vi "Configure Dialog.vi"(8 "Error In":errorcluster, 11 "Save SV to Library Msg in":refnum<class "Save SV to Library Msg.lvclass">) -> (0 "Error Out":errorcluster, 2 "OK?":bool, 3 "Save SV to Library Msg out":refnum<class "Save SV to Library Msg.lvclass">)   [LabVIEW 2014, in "CS++DSCManager.lvlib" / "Save SV to Library Msg.lvclass"]
doc: "This overrides of this dynamic dispatch VI open the frontpanel to set derived message attributes."
uses:
  Save SV to Library Msg.lvclass
  Save SV to Library Msg.lvclass/Save SV to Library Msg.ctl
panel:
  in  "OK":bool
  in  "Cancel":bool
  in  "Library Path":path
  in  "Shared Variables":refnum<k21>[](array[refnum])
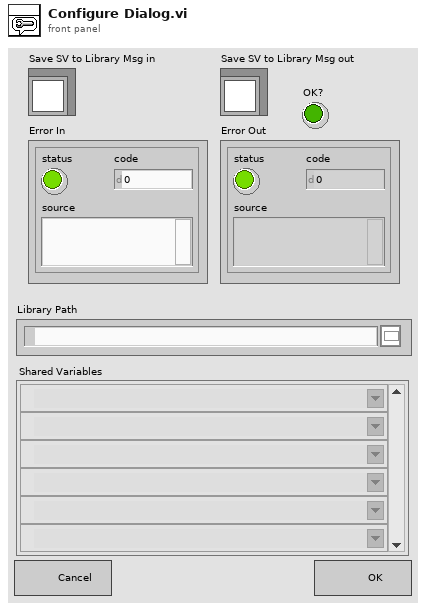
[diagram p1: front panel]
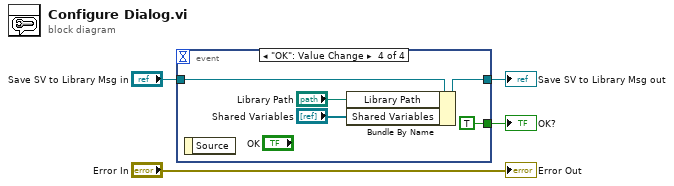
[diagram p0: block diagram]
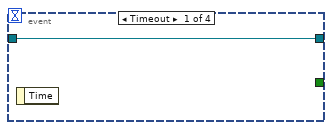
[diagram p2: hidden frame]
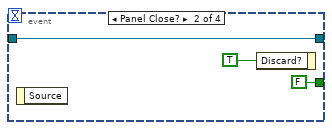
[diagram p3: hidden frame]
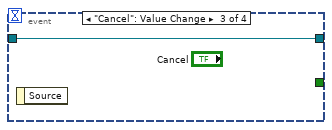
[diagram p4: hidden frame]
diagram:
  n1 = event shown="[3] \"OK\": Value Change" {
    selector: _ -> [_ _ _ _]
    dyn-events: _ -> [_ _ _ _]
    timeout: _ -> [_ _ _ _]
    tunnel: [w5 w6 w9 w13] -> w2
    tunnel: "Save SV to Library Msg in" -> [w5 w6 w9 w14]
    tunnel: [_ FALSE _ TRUE] -> w1
    event Timeout {
      n2 = event-data() -> ()  [unwired: 1 in, 1 out]
    }
    event Panel Close? {
      n3 = event-data() -> ()  [unwired: 1 in, 1 out]
      n4 = event-data("Discard?"=TRUE) -> ()  [unwired: 1 in, 1 out]
    }
    event "Cancel": Value Change {
      n5 = event-data() -> ()  [unwired: 1 in, 1 out]
    }
    event "OK": Value Change {
      n6 = event-data() -> ()  [unwired: 1 in, 1 out]
      n7 = Bundle By Name(cluster=w14, "Library Path"="Library Path", "Shared Variables"="Shared Variables") -> (w13:refnum<class "Save SV to Library Msg.lvclass">)
    }
  }
  "Save SV to Library Msg out" <- w2
  "OK?" <- w1
  "Error Out" <- "Error In"
